vi "Axis_Go Home.vi"(8 "error in":errorcluster, 11 "Axis Index":i32) -> (0 "error":errorcluster)   [LabVIEW 2019]
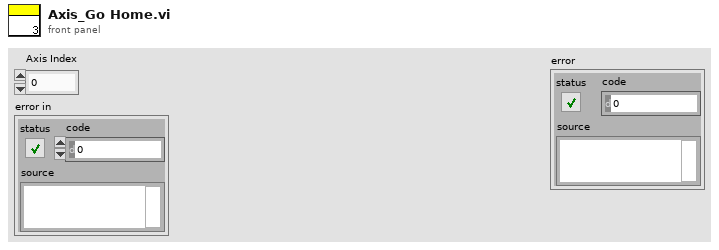
[diagram p1: front panel]
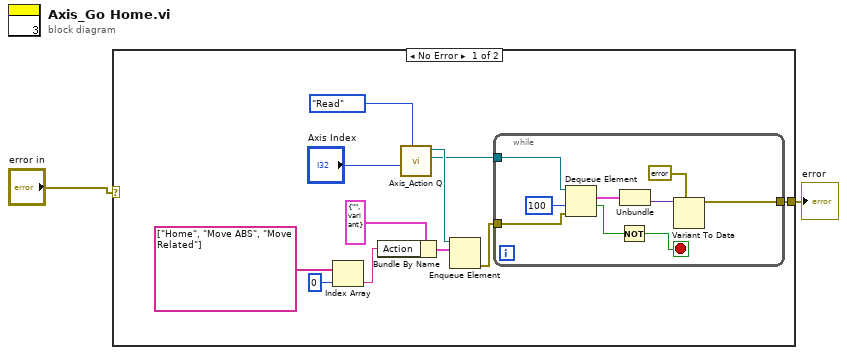
[diagram p0: block diagram]
diagram:
  n1 = case shown="No Error" "error in" {
    selector: "error in" -> [_ w23]
    tunnel: [w3 w23] -> w2
    frame No Error {
      n2 = Index Array(array=string[] ["Home", "Move ABS", "Move Related"], index=0) -> (element=w7:string)
      n3 = Bundle By Name(cluster=cluster{"Action":string, "Data":variant} {"Action"="", "Data"=variant} ("element"), "Action"=w7) -> (w8:cluster{"Action":string, "Data":variant})
      n4 = call "Axis_Action Q.vi"("Enum"=enum16{"Initial", "Write", "Read"}."Read", "Axis Index"="Axis Index") -> ("Axis ActFeedBackQ Out"=w5:refnum<queue>, "Axis ActQ Out"=w11:refnum<queue>)  [unwired: 7 in, 1 out]
      n5 = Enqueue Element(queue=w11, element=w8) -> (error out=w4:errorcluster)  [unwired: 2 in, 2 out]
      n6 = while {
        tunnel: w5 -> [w22]
        tunnel: w4 -> [w21]
        tunnel: [w14] -> w3
        stop <- w17 stop-if-true
        n7 = Dequeue Element(queue=w22, timeout in ms (-1)=100, error in (no error)=w21) -> (element=w19:cluster{"Action":string, "Data":variant}, timed out?=w18:bool)  [unwired: 2 out]
        n8 = Not(x=w18) -> (.not. x?=w17:bool)
        n9 = Unbundle(w19) -> ("Data"=w16:variant)  [unwired: 1 out]
        n10 = Variant To Data(type=errorcluster {"status"=FALSE, "code"=0, "source"=""} ("error constant"), Variant=w16) -> (data=w14:errorcluster)  [unwired: 1 in, 1 out]
      }
    }
    frame Error {
    }
  }
  "error" <- w2
